vi "manual_wait.vi"(8 "error in (no error)":errorcluster, 11 "data":variant) -> (0 "error out":errorcluster)   [LabVIEW 2015, in "lv-recipe-machine.lvlib" / "example_01.lvlib"]
doc: "manual_wait.vi will wait a given amount of time (or if not provided, a time between 0 and 2000ms) and output how much time it took."
uses:
  example_01.lvlib
  _controls/steps_actions.ctl
  _controls/steps_actions_data.ctl
  lv-recipe-machine.lvlib
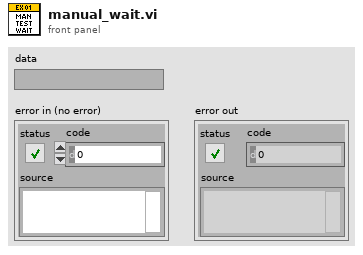
[diagram p1: front panel]
types:
  T1 = typedef "lv-recipe-machine.lvlib/example_01.lvlib/steps_actions_data.ctl" = cluster{"step_action":T2, "data":variant}
  T2 = typedef "lv-recipe-machine.lvlib/example_01.lvlib/steps_actions.ctl" = enum16{"<steps_actions>", "manual_random", "manual_comparison", "manual_wait", "auto_random", "auto_wait", "criteria_initialize", "criteria_count", "criteria_comparison", "transition_simple", "transition_count", "transition_comparison", "launch_wait", "<null>"}
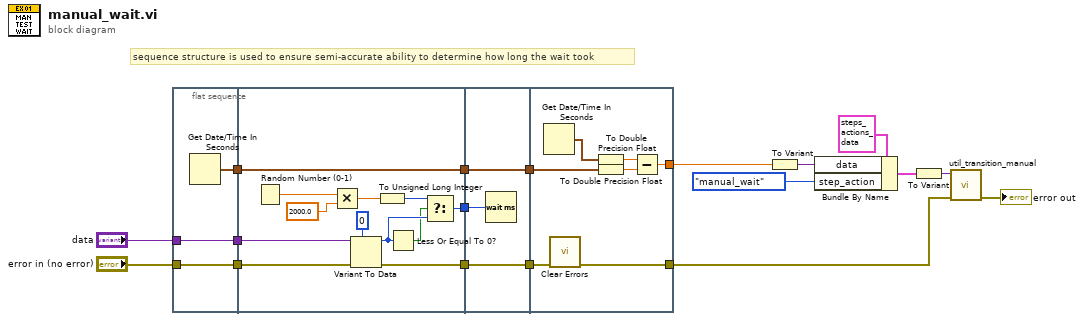
[diagram p0: block diagram]
diagram:
  # "sequence structure is used to ensure semi-accurate ability to determine how long the wait took"
  n1 = flat-sequence {
    tunnel: "data" -> [w21]
    tunnel: "error in (no error)" -> [w20]
    tunnel: [w21] -> w15
    tunnel: [w20] -> w14
    tunnel: [w19] -> w13
    tunnel: w15 -> [w26]
    tunnel: w14 -> [w27]
    tunnel: w13 -> [w33]
    tunnel: [w33] -> w12
    tunnel: [w25] -> w10
    tunnel: [w22] -> w5
    tunnel: w12 -> [w36]
    tunnel: [w36] -> w11
    tunnel: w10 -> [w35]
    tunnel: [w34] -> w6
    tunnel: w5 -> [w34]
    tunnel: w11 -> [w42]
    tunnel: [w41] -> w9
    tunnel: [w40] -> w7
    tunnel: w6 -> [w39]
    frame #0 {
      n2 = Get Date/Time In Seconds() -> (seconds since 1Jan1904=w19:timestamp)
    }
    frame #1 {
      n3 = Random Number (0-1)() -> (number: 0 to 1=w29:dbl)
      n4 = Multiply(x=w29, y=2000.0) -> (x*y=w31:dbl)
      n5 = Variant To Data(error in=w27, type=u32 0, Variant=w26) -> (data=w24:u32, error out=w22:errorcluster)
      n6 = To Unsigned Long Integer(number=w31) -> (unsigned 32bit integer=w32:u32)
      n7 = Less Or Equal To 0?(x=w24) -> (x <= 0?=w23:bool)
      n8 = Select(t=w32, s=w23, f=w24) -> (s? t:f=w25:u32)
    }
    frame #2 {
      n9 = Wait (ms)(milliseconds to wait=w35) -> ()  [unwired: 1 out]
    }
    frame #3 {
      n10 = Get Date/Time In Seconds() -> (seconds since 1Jan1904=w43:timestamp)
      n11 = call <vilib>:"Clear Errors.vi"("error in (no error)"=w39) -> ("error out"=w40:errorcluster)  [unwired: 5 in, 1 out]
      n12 = To Double Precision Float(number=w43) -> (double precision float=w38:dbl)
      n13 = To Double Precision Float(number=w42) -> (double precision float=w37:dbl)
      n14 = Subtract(x=w38, y=w37) -> (x-y=w41:dbl)
    }
  }
  n15 = To Variant(anything=w9) -> (Variant=w18:variant)
  n16 = Bundle By Name(cluster=T1 {"step_action"=enum."<steps_actions>", "data"=variant} ("step_data"), "data"=w18, "step_action"=steps_actions."manual_wait" ("manual_action")) -> (w8:T1)
  n17 = To Variant(anything=w8) -> (Variant=w4:variant)
  n18 = call "util_transition_manual.vi"("error in (no error)"=w7, "data"=w4) -> ("error out"=→"error out":errorcluster)  [unwired: 9 in]
